vi "update_rate_and_time.vi"(8 "error in (no error)":errorcluster) -> (0 "error out":errorcluster, 2 "time (ms)":u32, 3 "rate (Hz)":dbl)   [LabVIEW 2016, in "Lockin.DAQ.lvclass"]
uses:
  Lockin.DAQ.lvclass
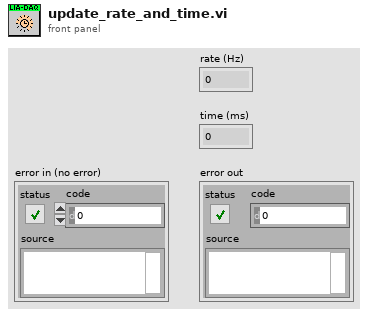
[diagram p1: front panel]
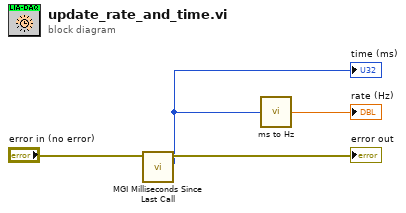
[diagram p0: block diagram]
diagram:
  n1 = call <userlib>:"MGI Milliseconds Since Last Call.vi"("Error In"="error in (no error)") -> ("ms"=w1:u32, "Error Out"=→"error out":errorcluster)  [unwired: 5 in]
  "time (ms)" <- w1
  n2 = call "ms to Hz.vi"("ms"=w1) -> ("Numeric"=→"rate (Hz)":dbl)
